vi "Write  Test_date to File.vi"(3 "error in":errorcluster, 4 "String":string, 5 "appended path":path) -> (0 "error out":errorcluster)   [LabVIEW 2012]
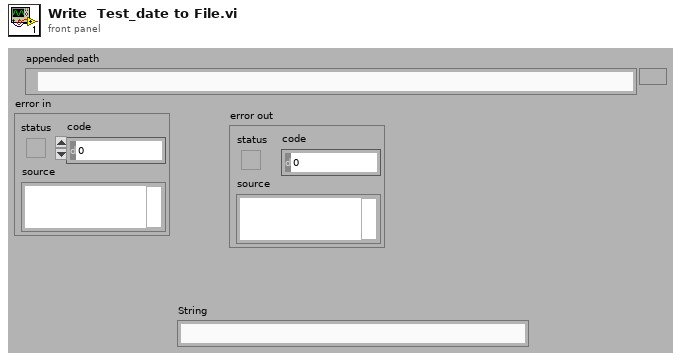
[diagram p1: front panel]
types:
  T1 = enum16{"open", "replace", "create", "open or create", "replace or create", "replace or create with confirmation"}
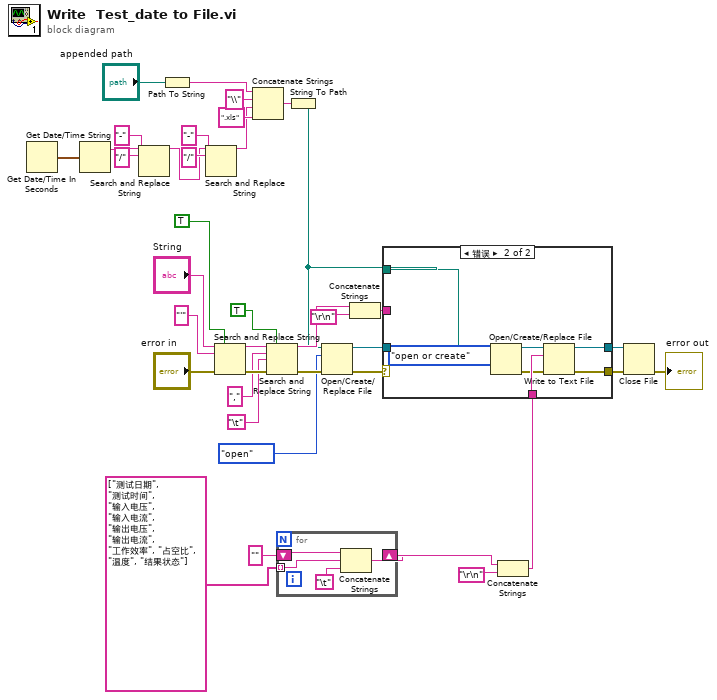
[diagram p0: block diagram]
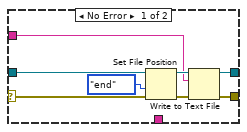
[diagram p2: hidden frame]
diagram:
  n1 = Get Date/Time In Seconds() -> (seconds since 1Jan1904=w14:timestamp)
  n2 = Get Date/Time String(seconds (now)=w14) -> (date string=w7:string)  [unwired: 2 in, 1 out]
  n3 = Search and Replace String(input string=w7, search string="/" ("子字符串(\"\")"), replace string="-" ("替换字符串(\"\")")) -> (result string=w2:string)  [unwired: 5 in, 3 out]
  n4 = Path To String(path="appended path") -> (string=w11:string)
  n5 = Search and Replace String(input string=w2, search string="/" ("子字符串(\"\")"), replace string="-" ("替换字符串(\"\")")) -> (result string=w1:string)  [unwired: 5 in, 3 out]
  n6 = Search and Replace String(replace all?=TRUE ("replace all? (F)"), input string="String", search string="'", error in="error in") -> (result string=w29:string, error out=w27:errorcluster)  [unwired: 4 in, 2 out]
  n7 = Concatenate Strings(w11, "\\" ("字符串"), w1, ".xls" ("字符串")) -> (w10:string)
  n8 = Search and Replace String(replace all?=TRUE ("replace all? (F)"), input string=w29, search string=",", replace string="\t", error in=w27) -> (result string=w26:string, error out=w22:errorcluster)  [unwired: 3 in, 2 out]
  n9 = for {
    shift-right: [w42] -> w16
    shift-left: "" -> [w41]
    tunnel: string[] ["测试日期", "测试时间", "输入电压", "输入电流", "输出电压", "输出电流", "工作效率", "占空比", "温度", "结果状态"] -> [w39] mode=indexing
    n10 = Concatenate Strings(w41, w39, "\t") -> (w42:string)
  }
  n11 = String To Path(string=w10) -> (path=w8:path)
  n12 = Open/Create/Replace File(file path (use dialog)=w8, error in=w22, operation (0:open)=T1."open" ("操作(0:open)")) -> (refnum out=w36:refnum<file>, error out=w35:errorcluster)  [unwired: 3 in, 1 out]
  n13 = Concatenate Strings(w26, "\r\n") -> (w21:string)
  n14 = Concatenate Strings(w16, "\r\n") -> (w15:string)
  n15 = case shown="错误" w35 {
    selector: w35 -> [w50 _]
    tunnel: w36 -> [w48 _]
    tunnel: [w45 w57] -> w37
    tunnel: [w44 w56] -> w38
    tunnel: w21 -> [w43 _]
    tunnel: w15 -> [_ w55]
    tunnel: w8 -> [_ w52]
    frame No Error {
      n16 = Set File Position(refnum=w48, from (0:start)=enum16{"start", "end", "current"}."end", error in=w50) -> (refnum out=w46:refnum<file>, error out=w47:errorcluster)  [unwired: 1 in]
      n17 = Write to Text File(file (use dialog)=w46, text=w43, error in=w47) -> (refnum out=w44:refnum<file>, error out=w45:errorcluster)  [unwired: 1 in, 1 out]
    }
    frame Error {
      n18 = Open/Create/Replace File(file path (use dialog)=w52, operation (0:open)=T1."open or create" ("操作(0:open)")) -> (refnum out=w54:refnum<file>, error out=w53:errorcluster)  [unwired: 4 in, 1 out]
      n19 = Write to Text File(file (use dialog)=w54, text=w55, error in=w53) -> (refnum out=w56:refnum<file>, error out=w57:errorcluster)  [unwired: 1 in, 1 out]
    }
  }
  n20 = Close File(refnum=w38, error in=w37) -> (error out=→"error out":errorcluster)  [unwired: 1 out]
